vi "Format Default Forecast Data.vi"(8 "error in":errorcluster, 11 "file path":path) -> (0 "error out":errorcluster, 1 "Data":dbl[](array[numeric]), 2 "dt (sec)":dbl, 3 "t0 (sec)":dbl)   [LabVIEW 2018, in "Generic Optimization Actor.lvlib" / "Generic Optimization.lvclass"]
uses:
  Generic Optimization.lvclass
  <vilib>/Utility/file.llb/Read Delimited Spreadsheet (DBL).vi
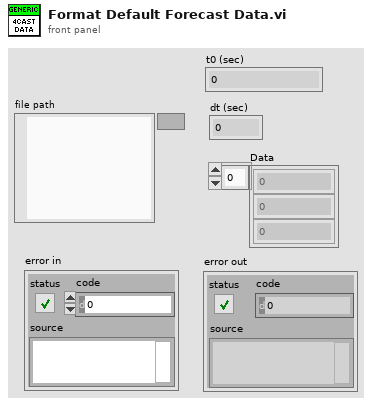
[diagram p1: front panel]
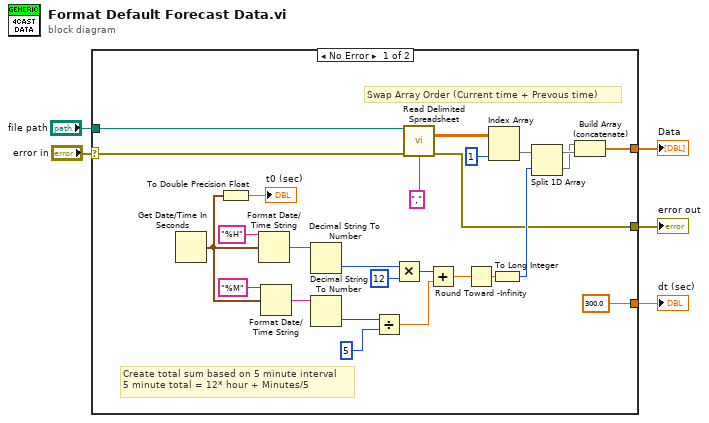
[diagram p0: block diagram]
diagram:
  n1 = case shown="No Error" "error in" {
    selector: "error in" -> [w7 w32]
    tunnel: [w30 _] -> w5
    tunnel: "file path" -> [w13 _]
    tunnel: [300.0 _] -> w3
    tunnel: [w6 w32] -> w1
    frame No Error {
      # "Swap Array Order (Current time + Prevous time)"
      # "Create total sum based on 5 minute interval\n5 minute total = 12* hour + Minutes/5"
      n2 = Get Date/Time In Seconds() -> (seconds since 1Jan1904=w8:timestamp)
      n3 = To Double Precision Float(number=w8) -> (double precision float=→"t0 (sec)":dbl)
      n4 = Format Date/Time String(time format string (%c)="%H", seconds (now)=w8) -> (date/time string=w16:string)  [unwired: 1 in]
      n5 = Format Date/Time String(time format string (%c)="%M", seconds (now)=w8) -> (date/time string=w19:string)  [unwired: 1 in]
      n6 = Decimal String To Number(string=w16) -> (number=w17:i32)  [unwired: 2 in, 1 out]
      n7 = Decimal String To Number(string=w19) -> (number=w20:i32)  [unwired: 2 in, 1 out]
      n8 = Divide(x=w20, y=5) -> (x/y=w22:dbl)
      n9 = Multiply(x=w17, y=12) -> (x*y=w23:i32)
      n10 = call-poly <vilib>:"Read Delimited Spreadsheet.vi"("file path (dialog if empty)"=w13, "error in (no error)"=w7, "delimiter (\\t)"="," ("delimiter (\\t)")) -> ("all rows"=w26:dbl[][], "error out"=w6:errorcluster)  [unwired: 7 in, 4 out]
      n11 = Add(x=w23, y=w22) -> (x+y=w24:dbl)
      n12 = Round Toward -Infinity(1:w24) -> (0:w31:dbl)
      n13 = Index Array(array=w26, index (col)=1 ("disabled index (col)")) -> (element=w28:dbl[])  [unwired: 1 in]
      n14 = To Long Integer(number=w31) -> (32bit integer=w11:i32)
      n15 = Split 1D Array(array=w28, index=w11) -> (first subarray=w29:dbl[], second subarray=w27:dbl[])
      n16 = Build Array (concatenate)(w27, w29) -> (w30:dbl[])
    }
    frame Error {
    }
  }
  "Data" <- w5
  "dt (sec)" <- w3
  "error out" <- w1
